vi "Available Roles.vi"(8 "error in (no error)":errorcluster, 11 "Roles API in":refnum<class "Roles API.lvclass">) -> (0 "error out":errorcluster, 2 "Roles Available":string[](array[string]), 3 "Roles API out":refnum<class "Roles API.lvclass">)   [LabVIEW 2020, in "Volatus.lvlib" / "Roles API.lvclass"]
uses:
  Roles API.lvclass
  Roles API.lvclass/Roles API.ctl
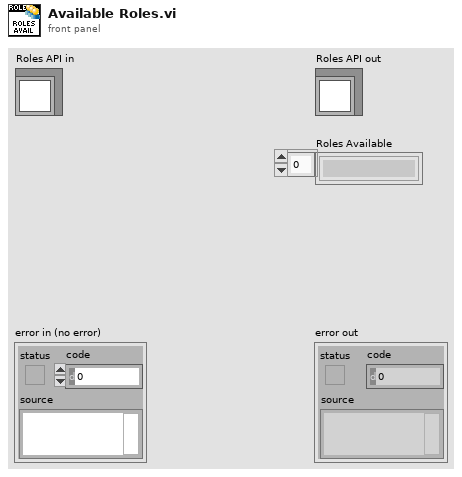
[diagram p1: front panel]
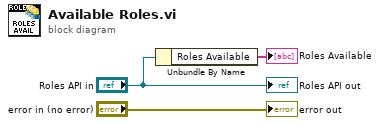
[diagram p0: block diagram]
diagram:
  n1 = Unbundle By Name("Roles API in") -> ("Roles Available"=→"Roles Available":string[])
  "error out" <- "error in (no error)"
  "Roles API out" <- "Roles API in"
